vi "Calculate DC measurement scalar results.vi"(11 "DC measurement results":T1) -> (3 "output cluster":T1)   [LabVIEW 2021, in "Linearity_ADC.lvlib"]
uses:
  Linearity_ADC.lvlib
  Measurement Results.ctl
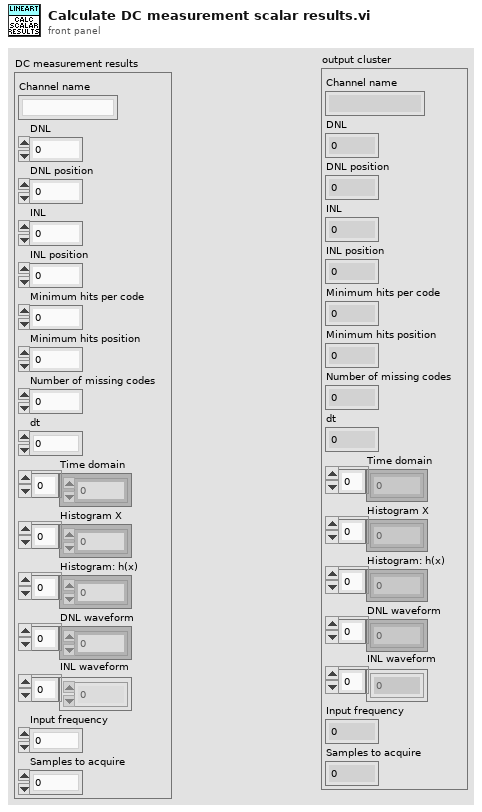
[diagram p1: front panel]
types:
  T1 = typedef "Linearity_ADC.lvlib/Measurement Results.ctl" = cluster{"Channel name":string, "DNL":dbl, "DNL position":i32, "INL":dbl, "INL position":i32, "Minimum hits per code":i32, "Minimum hits position":i32, "Number of missing codes":i32, "dt":dbl, "Time domain":dbl[], "Histogram X":dbl[], "Histogram: h(x)":i32[], "DNL waveform":dbl[], "INL waveform":dbl[], "Input frequency":dbl, "Samples to acquire":u32}
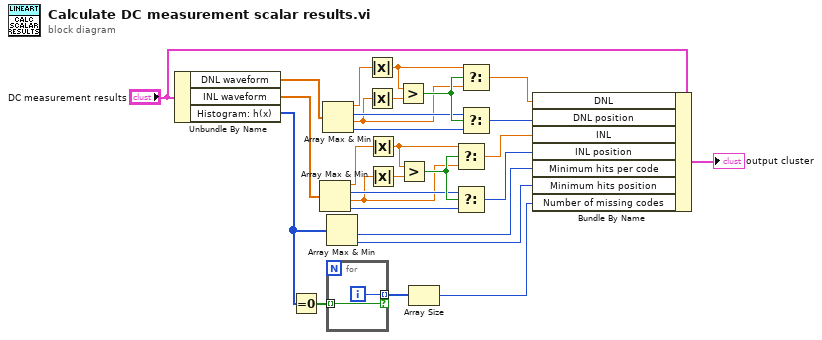
[diagram p0: block diagram]
diagram:
  n1 = Unbundle By Name("DC measurement results") -> ("DNL waveform"=w20:dbl[], "INL waveform"=w19:dbl[], "Histogram: h(x)"=w26:i32[])
  n2 = Equal To 0?(x=w26) -> (x = 0?=w25:bool[])
  n3 = Array Max & Min(array=w19) -> (max value=w18:dbl, max index (indices)=w4:i32, min value=w1:dbl, min index (indices)=w5:i32)
  n4 = Array Max & Min(array=w20) -> (max value=w14:dbl, max index (indices)=w8:i32, min value=w2:dbl, min index (indices)=w7:i32)
  n5 = Array Max & Min(array=w26) -> (min value=w28:i32, min index (indices)=w27:i32)  [unwired: 2 out]
  n6 = for {
    tunnel: w25 -> [w30] mode=indexing
    tunnel: [w29] -> w23 mode=indexing if=w30
    i -> [w29]
  }
  n7 = Absolute Value(x=w14) -> (abs(x)=w12:dbl)
  n8 = Absolute Value(x=w2) -> (abs(x)=w11:dbl)
  n9 = Absolute Value(x=w18) -> (abs(x)=w17:dbl)
  n10 = Absolute Value(x=w1) -> (abs(x)=w16:dbl)
  n11 = Greater?(x=w12, y=w11) -> (0:w13:bool)
  n12 = Greater?(x=w17, y=w16) -> (0:w6:bool)
  n13 = Array Size(array=w23) -> (size(s)=w24:i32)
  n14 = Select(t=w17, s=w6, f=w1) -> (s? t:f=w15:dbl)
  n15 = Select(t=w4, s=w6, f=w5) -> (s? t:f=w3:i32)
  n16 = Select(t=w12, s=w13, f=w2) -> (s? t:f=w10:dbl)
  n17 = Select(t=w8, s=w13, f=w7) -> (s? t:f=w9:i32)
  n18 = Bundle By Name(cluster="DC measurement results", "DNL"=w10, "DNL position"=w9, "INL"=w15, "INL position"=w3, "Minimum hits per code"=w28, "Minimum hits position"=w27, "Number of missing codes"=w24) -> (→"output cluster":T1)
